vi "FTW-Regex-ReplaceAndReturn.vi"(0 "String":string, 5 "Search for (Regular Expression)":string, 7 "Replace with":string, 11 "error in":errorcluster) -> (4 "String out":string, 6 "Original Match (replaced)":string, 8 "Submatches":string[](array[string]), 10 "Match Found?":bool, 15 "error out":errorcluster)   [LabVIEW 2015]
uses:
  FTW-Regex-Execute.vi
  error/FTW-ERR-ThrowGenericError.vi
  error/FTW-ERR-ThrowError.vi
  error/FTW-ERR-CallChain.vi
  error/FTW-ERR-NoErrorConstant.vi
  string/FTW-STR-ReplaceWhitespace.vi
  string/FTW-STR-Array-Delimit.vi
  error/FTW-ERR-Clear.vi
  FTW-Regex-ReplaceAll.vi
  FTW-Regex-Destroy.vi
  lib/FTW-KernelFilepath.vi
  FTW-Regex-Construct.vi
panel:
  in  "Starting Offset":i32
  # "Inputs"
  # "Outputs"
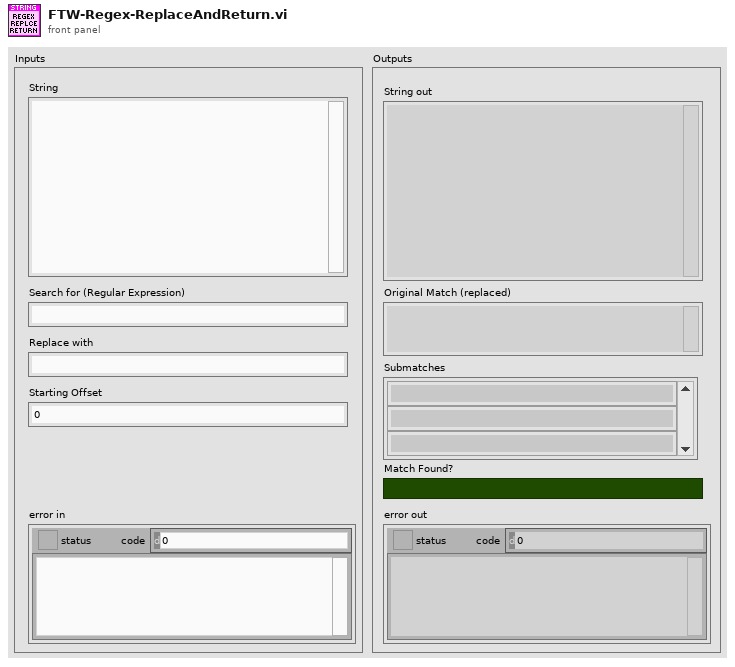
[diagram p1: front panel]
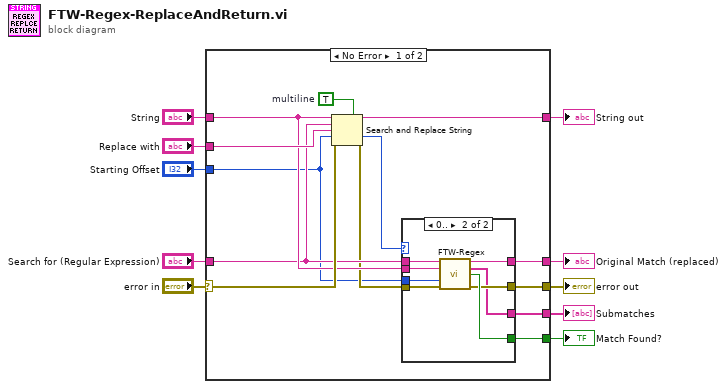
[diagram p0: block diagram]
diagram:
  n1 = case shown="No Error" "error in" {
    selector: "error in" -> [w22 w35]
    tunnel: [w13 w35] -> w10
    tunnel: "String" -> [w19 w34]
    tunnel: [w23 w34] -> w7
    tunnel: "Replace with" -> [w21 _]
    tunnel: "Search for (Regular Expression)" -> [w16 _]
    tunnel: "Starting Offset" -> [w12 _]
    tunnel: [w18 _] -> w3
    tunnel: [w15 _] -> w2
    tunnel: [w11 _] -> w1
    frame No Error {
      w20 = TRUE  # multiline
      n2 = Search and Replace String(multiline?=w20, input string=w19, search string=w16, replace string=w21, offset=w12, error in=w22) -> (result string=w23:string, offset past replacement=w17:i32, error out=w14:errorcluster)  [unwired: 2 in, 1 out]
      n3 = case shown="0.." w17 {
        tunnel: w19 -> [_ w32]
        tunnel: [w24 w31] -> w18
        tunnel: w16 -> [w24 w33]
        tunnel: [_ w30] -> w15
        tunnel: w14 -> [w25 w29]
        tunnel: [w25 w28] -> w13
        tunnel: w12 -> [_ w27]
        tunnel: [_ w26] -> w11
        frame ..-1 {
        }
        frame 0.. {
          n4 = call "FTW-Regex.vi"("Regular Expression"=w33, "Input String"=w32, "Starting Offset"=w27, "error in"=w29) -> ("Match"=w31:string, "Submatches"=w26:string[], "Match Found?"=w30:bool, "error out"=w28:errorcluster)  [unwired: 7 in, 1 out]
        }
      }
    }
    frame Error {
    }
  }
  "error out" <- w10
  "String out" <- w7
  "Original Match (replaced)" <- w3
  "Match Found?" <- w2
  "Submatches" <- w1
